vi "Remote Calibration FPGA Loop.vi"   [LabVIEW 2014]
uses:
  Remote Calibration Typedef.ctl
  MC State Machine.lvsc/State.ctl
  <vilib>/FPGAPlugInAG/sbRIO-9626/niLvFpga_Open_sbRIO-9626.vi
  <vilib>/rvi/interface/common/dynamic/niFpgaDynamicAddResources.vi
  <vilib>/Utility/error.llb/Error Cluster From Error Code.vi
  <vilib>/rvi/errors/niLvFpgaAdjustHostInterfaceError.vi
  Global Data.vi
  <vilib>/FPGAPlugInAG/Dynamic/niLvFpga_Close_Dynamic.vi
  <vilib>/rvi/interface/nirviOpenFPGA/nirviOpenFPGA.xnode
  FPGA Bitfiles/FormulaElectric2_FPGATarget_FPGA_8a5J0mMac2U.lvbitx
  <vilib>/rvi/interface/nirviReadWriteControl/nirviReadWriteControl.xnode
  <vilib>/rvi/interface/nirviCloseFPGA/nirviCloseFPGA.xnode
  <vilib>/rvi/interface/Simulation/niFpgaSimulationCallBeginRW.vi
  MC State Machine.lvsc
  NiFpgaLv.dll
types:
  T1 = typedef "MC State Machine.lvsc/State.ctl" = enum16{"NI.SC.Initial", "NI.SC.History", "NI.SC.ShallowHistory", "NI.SC.Terminal", "Let Current Drop then Disable AIR's", "Enabled", "Disabled"}
  T2 = typedef "Remote Calibration Typedef.ctl" = cluster{"Rear BP Scaling Factor":fxp<+,11,11>, "Front BP Scaling Factor":fxp<+,11,11>, "Rear BP Offset (V)":fxp<+/-,26,5>, "Front BP Offset":fxp<+/-,26,5>, "Throttle 2 Max":fxp<+,16,4>, "Throttle 2 Min":fxp<+,16,4>, "Throttle 1 Max":fxp<+,16,4>, "Throttle 1 Min":fxp<+,16,4>, "MC Update Period (ms)":u32, "Regen Mult.":dbl, "Zero Torque %":dbl, "Torque Mult.":dbl, "Activation Brake Pressure":dbl}
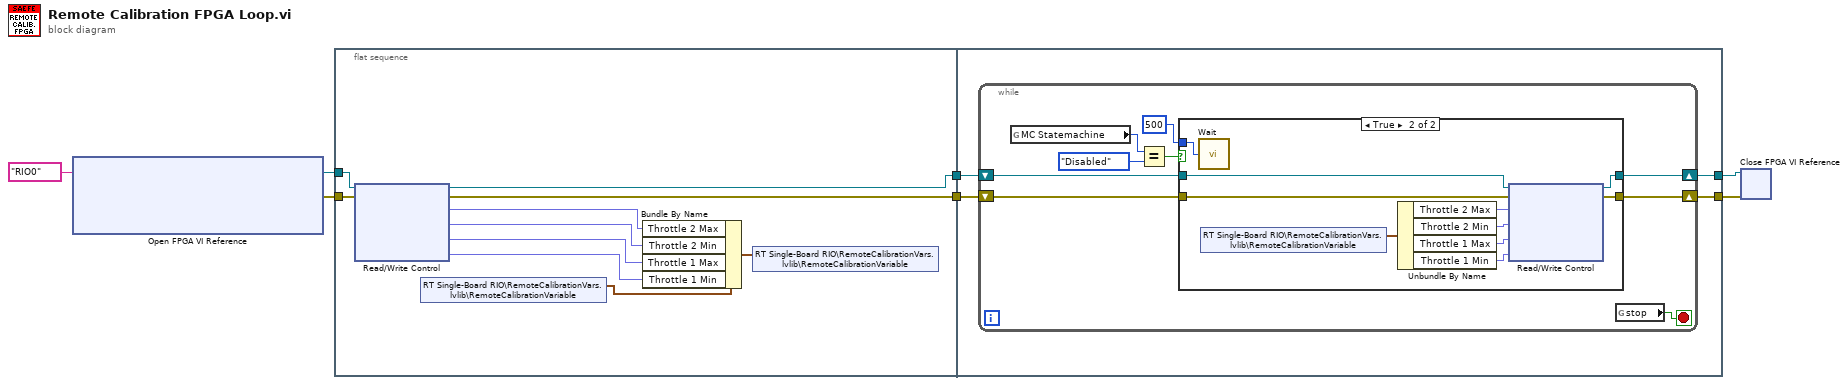
[diagram p0: block diagram]
diagram:
  n1 = xnode "Open FPGA VI Reference"("resource name"=tag "RIO0") -> ("FPGA VI Reference Out"=w7:refnum<k20>, "error out"=w6:errorcluster)  [unwired: 1 in]
  n2 = flat-sequence {
    tunnel: w7 -> [w15]
    tunnel: w6 -> [w14]
    tunnel: [w9] -> w5
    tunnel: [w8] -> w4
    tunnel: w5 -> [w21]
    tunnel: w4 -> [w20]
    tunnel: [w19] -> w3
    tunnel: [w18] -> w2
    frame #0 {
      n3 = xnode "Read/Write Control"("FPGA VI Reference In"=w15, "error in"=w14) -> ("FPGA VI Reference Out"=w9:refnum<k20>, "error out"=w8:errorcluster, "Throttle 2 Max"=w13:fxp<+,16,4>, "Throttle 2 Min"=w12:fxp<+,16,4>, "Throttle 1 Max"=w11:fxp<+,16,4>, "Throttle 1 Min"=w10:fxp<+,16,4>)
      n4 = shared-variable "RT Single-Board RIO\\RemoteCalibrationVars.lvlib\\RemoteCalibrationVariable"() -> (w16:T2)  [unwired: 1 in, 1 out]
      n5 = Bundle By Name(cluster=w16, "Throttle 2 Max"=w13, "Throttle 2 Min"=w12, "Throttle 1 Max"=w11, "Throttle 1 Min"=w10) -> (w17:T2)
      n6 = shared-variable "RT Single-Board RIO\\RemoteCalibrationVars.lvlib\\RemoteCalibrationVariable"(w17) -> ()  [unwired: 1 in, 1 out]
    }
    frame #1 {
      n7 = while {
        shift-right: [w26] -> w19
        shift-left: w21 -> [w28]
        shift-right: [w25] -> w18
        shift-left: w20 -> [w27]
        stop <- w30 stop-if-true
        n8 = global read "Global Data.vi" "MC Statemachine"() -> (w24:T1)
        n9 = Equal?(x=w24, y=State."Disabled") -> (x = y?=w22:bool)
        n10 = case shown="True" w22 {
          tunnel: u32 500 ("Count(mSec)") -> [_ w42]
          tunnel: w28 -> [w32 w41]
          tunnel: w27 -> [w31 w40]
          tunnel: [w32 w39] -> w26
          tunnel: [w31 w38] -> w25
          frame False {
          }
          frame True {
            n11 = call "Wait"("Count(mSec)"=w42) -> ()  [unwired: 1 out]
            n12 = shared-variable "RT Single-Board RIO\\RemoteCalibrationVars.lvlib\\RemoteCalibrationVariable"() -> (w37:T2)  [unwired: 1 in, 1 out]
            n13 = Unbundle By Name(w37) -> ("Throttle 2 Max"=w36:fxp<+,16,4>, "Throttle 2 Min"=w35:fxp<+,16,4>, "Throttle 1 Max"=w34:fxp<+,16,4>, "Throttle 1 Min"=w33:fxp<+,16,4>)
            n14 = xnode "Read/Write Control"("FPGA VI Reference In"=w41, "error in"=w40, "Throttle 2 Max"=w36, "Throttle 2 Min"=w35, "Throttle 1 Max"=w34, "Throttle 1 Min"=w33) -> ("FPGA VI Reference Out"=w39:refnum<k20>, "error out"=w38:errorcluster)
          }
        }
        n15 = global read "Global Data.vi" "stop"() -> (w30:bool)
      }
    }
  }
  n16 = xnode "Close FPGA VI Reference"("FPGA VI Reference In"=w3, "error in"=w2) -> ()  [unwired: 1 out]
